vi "Get Attributes.vi"(8 "error in (no error)":errorcluster, 11 "For Loop Dialog in":refnum<class "For Loop Dialog.lvclass">) -> (0 "error out":errorcluster, 3 "For Loop Dialog out":refnum<class "For Loop Dialog.lvclass">)   [LabVIEW 2017, in "For Loop Dialog.lvclass"]
uses:
  For Loop Dialog.lvclass
  ITest Executive Builder Dialog/ITest Executive Builder Dialog.lvclass
  <vilib>/gpm_packages/@cs/test-executive/Source/Test Executive/TestExecutive Ref/TestExecutive Ref.lvclass
  bd3c3d9a-c639-4d3a-a825-43e3a07e4ab5.vi
  15e9dcfe-feeb-47cb-bd1a-ededd49e8d7b.vi
  C:/Users/huijun.guo/Desktop/composed-test-executive-builder/Source/Test Executive Builder Dialogs/ITest Executive Builder Dialog/ITest Executive Builder Dialog.lvclass
  C:/Program Files/National Instruments/LabVIEW 2017/vi.lib/gpm_packages/@cs/popup-viewmanager/Source/Popup ViewManager/Popup ViewManager.lvclass
  C:/Program Files/National Instruments/LabVIEW 2017/vi.lib/gpm_packages/@cs/mva-dialogbox/source/IDialogBox/IDialogBox/IDialogBox.lvclass
  C:/Program Files/National Instruments/LabVIEW 2017/vi.lib/gpm_packages/@cs/mva-viewable/Source/IViewable/IViewable/IViewable.lvclass
  C:/Program Files/National Instruments/LabVIEW 2017/vi.lib/gpm_packages/@cs/mva-viewable/Source/ActorEvents/IEventAggregator/IEventAggregator.lvclass
  C:/Program Files/National Instruments/LabVIEW 2017/vi.lib/gpm_packages/@cs/mva-core/Source/IObserver/IObserver/IObserver.lvclass
  C:/Program Files/National Instruments/LabVIEW 2017/vi.lib/ActorFramework/Actor/Actor.lvclass
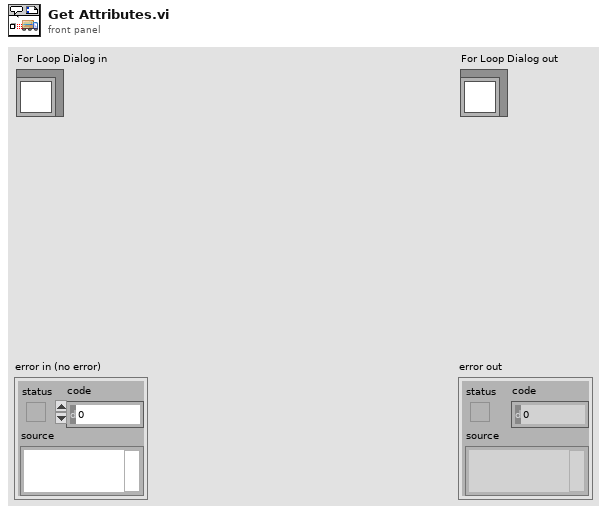
[diagram p1: front panel]
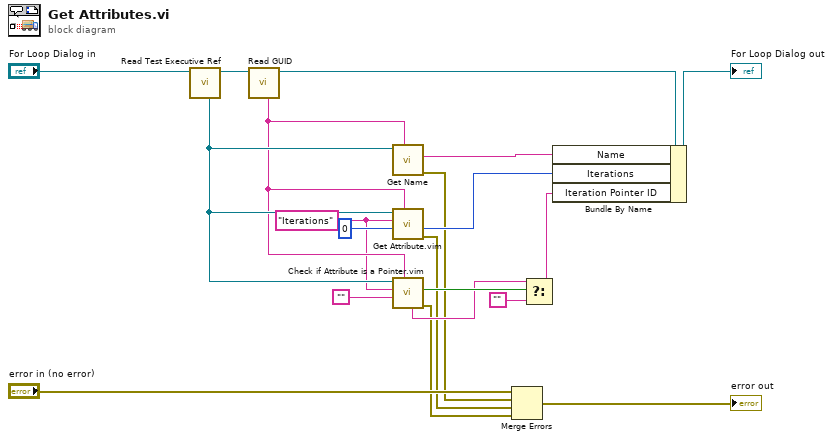
[diagram p0: block diagram]
diagram:
  w11 = "Iterations" ("Attribute Name")
  n1 = call "Read Test Executive Ref.vi"("ITest Executive Builder Dialog in"="For Loop Dialog in") -> ("ITest Executive Builder Dialog out"=w19:refnum<class "For Loop Dialog.lvclass">, "Test Executive Ref"=w13:refnum<data-value>)  [unwired: 9 in]
  n2 = call "Read GUID.vi"("ITest Executive Builder Dialog in"=w19) -> ("ITest Executive Builder Dialog out"=w17:refnum<class "For Loop Dialog.lvclass">, "GUID"=w12:string)  [unwired: 9 in]
  n3 = call <vilib>:"Get Name.vi"("Unique ID"=w12, "Test Executive Ref"=w13) -> ("error out"=w1:errorcluster, "Name"=w18:string)  [unwired: 5 in, 3 out]
  n4 = call "Get Attribute.vim"("ID"=w12, "Type"=0, "Attribute Name"=w11, "Test Executive Ref"=w13) -> ("error out"=w2:errorcluster, "Attribute"=w14:i32)  [unwired: 3 in, 3 out]
  n5 = call "Check if Attribute is a Pointer.vim"("ID"=w12, "Type"="", "Attribute Name"=w11, "Test Executive Ref"=w13) -> ("error out"=w3:errorcluster, "Pointer?"=w9:bool, "Pointer ID"=w8:string)  [unwired: 3 in, 2 out]
  n6 = Merge Errors("error in (no error)", w1, w2, w3) -> (→"error out":errorcluster)
  n7 = Select(t=w8, s=w9, f="") -> (s? t:f=w6:string)
  n8 = Bundle By Name(cluster=w17, "Name"=w18, "Iterations"=w14, "Iteration Pointer ID"=w6) -> (→"For Loop Dialog out":refnum<class "For Loop Dialog.lvclass">)
